vi "V2P4_Test_R0.vi"() -> ()   [LabVIEW 2011]
uses:
  <vilib>/Instr/_visa.llb/VISA Set IO Buffer Mask.ctl
  <vilib>/Instr/_visa.llb/VISA Configure Serial Port (Instr).vi
panel:
  out "Sweep Metric":u32(graph)
  out "Pass":u32
  out "Frame ms":u32
  out "Index":u16
  out "Bytes at Port":u32
  out "Point ms":u32
  in  "Exit":bool
  out "error out":errorcluster
  in  "VISA resource name":refnum<visa-resource-name>="COM4"
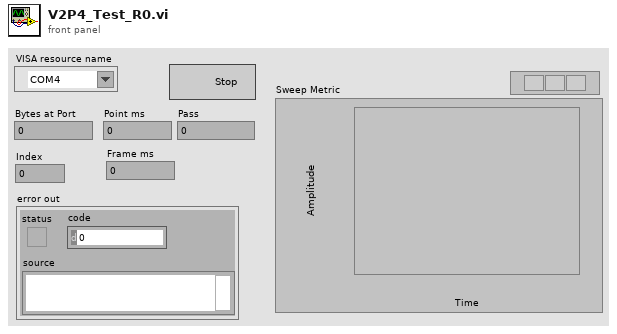
[diagram p1: front panel]
types:
  T1 = typedef "VISA Set IO Buffer Mask.ctl" = u16
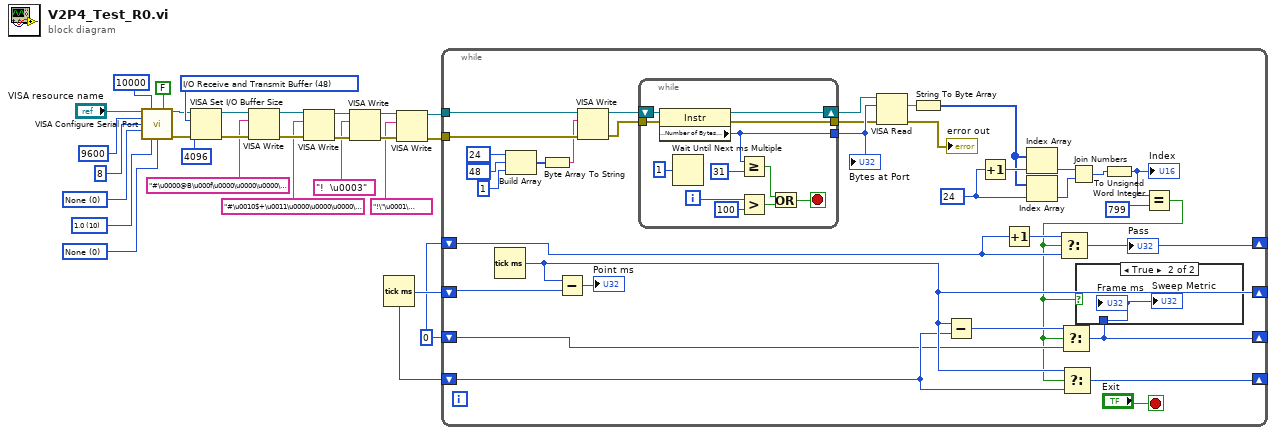
[diagram p0: block diagram]
diagram:
  w11 = u32 0
  w28 = u16 10 items=["1.0"=10, "1.5"=15, "2.0"=20] ("stop bits (10: 1 bit)")
  w26 = u16 0 items=["None", "Odd", "Even", "Mark", "Space"] ("parity")
  w27 = u16 0 items=["None"=0, "XON/XOFF"=1, "RTS/CTS"=2, "DTR/DSR"=4] ("flow control")
  w24 = T1 48 items=["I/O Receive Buffer"=16, "I/O Transmit Buffer"=32, "I/O Receive and Transmit Buffer"=48] ("Mask")
  n1 = call-poly "VISA Configure Serial Port"("VISA resource name"="VISA resource name", "timeout (10sec)"=u32 10000, "Enable Termination\nChar (T)"=FALSE ("Enable Termination Char (T)"), "baud rate (9600)"=u32 9600 ("baud rate"), "data bits (8)"=u16 8 ("data bits"), "parity (0:none)"=w26, "stop bits (10: 1 bit)"=w28, "flow control (0:none)"=w27) -> ("VISA resource name out"=w19:refnum<visa-resource-name>, "error out"=w17:errorcluster)  [unwired: 1 in, 5 out]
  n2 = VISA Set I/O Buffer Size(VISA resource name=w19, mask (16)=w24, size (4096)=u32 4096 ("Bufsize"), error in (no error)=w17) -> (VISA resource name out=w16:refnum<visa-resource-name>, error out=w15:errorcluster)
  n3 = VISA Write(VISA resource name=w16, write buffer="#\u0000@B\u000f\u0000\u0000\u0000\u0000\u0000" ("string 2"), error in (no error)=w15) -> (VISA resource name out=w12:refnum<visa-resource-name>, error out=w13:errorcluster)  [unwired: 1 out]
  n4 = VISA Write(VISA resource name=w12, write buffer="#\u0010$+\u0011\u0000\u0000\u0000\u0000\u0000" ("string 3"), error in (no error)=w13) -> (VISA resource name out=w8:refnum<visa-resource-name>, error out=w7:errorcluster)  [unwired: 1 out]
  n5 = VISA Write(VISA resource name=w8, write buffer="!  \u0003" ("string"), error in (no error)=w7) -> (VISA resource name out=w9:refnum<visa-resource-name>, error out=w10:errorcluster)  [unwired: 1 out]
  n6 = Tick Count (ms)() -> (millisecond timer value=w14:u32)
  n7 = VISA Write(VISA resource name=w9, write buffer="!\"\u0001\u0000" ("string 4"), error in (no error)=w10) -> (VISA resource name out=w5:refnum<visa-resource-name>, error out=w6:errorcluster)  [unwired: 1 out]
  n8 = while {
    tunnel: w5 -> [w63]
    tunnel: w6 -> [w62]
    shift-right: [w39] -> _
    shift-left: w14 -> [w51]
    shift-right: [w38] -> _
    shift-left: w14 -> [w37]
    shift-right: [w29] -> _
    shift-left: w11 -> [w36]
    shift-right: [w33] -> _
    shift-left: w11 -> [w32]
    stop <- "Exit" stop-if-true
    w42 = 24 ("index")
    n9 = Tick Count (ms)() -> (millisecond timer value=w39:u32)
    n10 = Build Array(u8 24 ("ReadFIFO"), u8 48 ("Address"), u8 1 ("element")) -> (w58:u8[])
    n11 = Byte Array To String(unsigned byte array=w58) -> (string=w59:string)
    n12 = Subtract(x=w39, y=w51) -> (x-y=→"Point ms":u32)
    n13 = VISA Write(VISA resource name=w63, write buffer=w59, error in (no error)=w62) -> (VISA resource name out=w54:refnum<visa-resource-name>, error out=w48:errorcluster)  [unwired: 1 out]
    n14 = while {
      tunnel: [w73] -> w57
      tunnel: [w76] -> w56
      shift-right: [w74] -> w53
      shift-left: w54 -> [w75]
      tunnel: w48 -> [w71]
      i -> [w69]
      stop <- w66 stop-if-true
      n15 = property class="Instr"(reference=w75, error in=w71) -> (reference out=w74:refnum<visa-resource-name>, error out=w76:errorcluster, "Serial Settings:Number of Bytes at Serial Port"=w73:u32)
      n16 = Wait Until Next ms Multiple(millisecond multiple=u32 1) -> ()  [unwired: 1 out]
      n17 = Greater Or Equal?(x=w73, y=u32 31) -> (x >= y?=w67:bool)
      n18 = Greater?(x=w69, y=100) -> (0:w68:bool)
      n19 = Or(x=w67, y=w68) -> (x .or. y?=w66:bool)
    }
    "Bytes at Port" <- w57
    n20 = VISA Read(VISA resource name=w53, byte count=w57, error in (no error)=w56) -> (read buffer=w55:string, error out=→"error out":errorcluster)  [unwired: 2 out]
    n21 = String To Byte Array(string=w55) -> (unsigned byte array=w41:u8[])
    n22 = Subtract(x=w39, y=w37) -> (x-y=w40:u32)
    n23 = Increment(x=w42) -> (x+1=w45:i32)
    n24 = Increment(x=w32) -> (x+1=w31:u32)
    n25 = Index Array(array=w41, index=w45) -> (element=w43:u8)
    n26 = Index Array(array=w41, index=w42) -> (element=w44:u8)
    n27 = Join Numbers(hi=w43, lo=w44) -> ((hi.lo)=w46:u16)
    n28 = To Unsigned Word Integer(number=w46) -> (unsigned 16bit integer=w35:u16)
    "Index" <- w35
    n29 = Equal?(x=w35, y=u16 799 ("SweepPoints")) -> (x = y?=w30:bool)
    n30 = Select(t=w31, s=w30, f=w32) -> (s? t:f=w33:u32)
    "Pass" <- w33
    n31 = Select(t=w40, s=w30, f=w36) -> (s? t:f=w29:u32)
    n32 = Select(t=w39, s=w30, f=w37) -> (s? t:f=w38:u32)
    n33 = case shown="True" w30 {
      tunnel: w29 -> [_ w64]
      frame False {
      }
      frame True {
        "Sweep Metric" <- w64
        "Frame ms" <- w64
      }
    }
  }
